vi "Get SMO HELP.vi"(8 "error in (no error)":errorcluster, 10 "Command":string, 11 "Inst.FP in":refnum<class "Inst.FP.lvclass">) -> (0 "error out":errorcluster, 2 "help cluster":T1, 3 "Inst.FP out":refnum<class "Inst.FP.lvclass">)   [LabVIEW 2019, in "Inst.FP.lvclass"]
uses:
  Inst.FP.lvclass
  <userlib>/LevyLab/Instrument Framework/subsystems/Help/typedefs/Help--cluster.ctl
  Typedefs/Inst.FP.Commands--Enum.ctl
  Typedefs/Inst.FP.pushButton--Cluster.ctl
  Typedefs/Inst.FP.Buttons--Enum.ctl
  Typedefs/Inst.FP.setMode--Cluster.ctl
  Typedefs/Inst.FP.Modes--Enum.ctl
  Typedefs/Inst.FP.getMode--Cluster.ctl
  <userlib>/LevyLab/Instrument Framework/Instrument Types/Cryostat/Instrument.Cryostat.lvclass
  <userlib>/LevyLab/Instrument Framework/subsystems/Help/Help.lvclass
  <userlib>/LevyLab/Instrument Framework/Instrument/Typedefs/Instrument.Commands--Enum.ctl
  <userlib>/LevyLab/Instrument Framework/Instrument/Instrument.lvclass
  <userlib>/LevyLab/Instrument Framework/Instrument/Typedefs/Instrument.IDN--cluster.ctl
  <vilib>/PRIrvin/JSON-Schema/JSON-Schema.lvlib
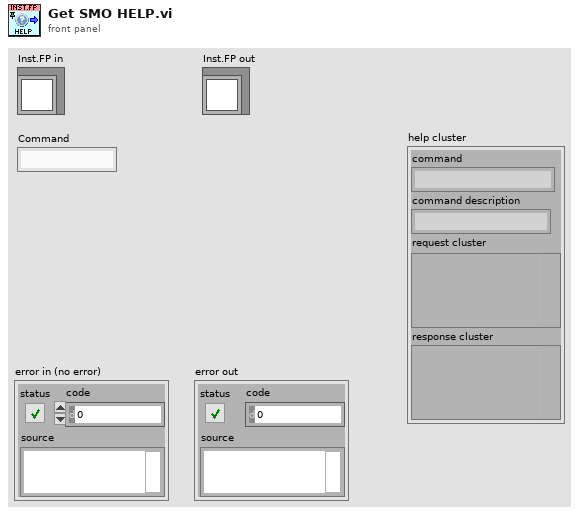
[diagram p1: front panel]
types:
  T1 = typedef "Instrument.lvlib/Help.lvclass/Help--cluster.ctl" = cluster{"command":string, "command description":string, "request cluster":variant, "response cluster":variant}
  T2 = typedef "Inst.FP.lvclass/Inst.FP.pushButton--Cluster.ctl" = cluster{"Button":T3}
  T3 = typedef "Inst.FP.lvclass/Inst.FP.Buttons--Enum.ctl" = enum16{"Start", "3He", "4He", "Normal", "Recovery", "Auto", "LED Test", "Reset"}
  T4 = typedef "Inst.FP.lvclass/Inst.FP.setMode--Cluster.ctl" = cluster{"Mode":T5}
  T5 = typedef "Inst.FP.lvclass/Inst.FP.Modes--Enum.ctl" = enum16{"AUTO MODE OFF", "START", "CONDENSING 3He", "CONDENSING 4He", "NORMAL CIRCULATION", "RECOVERY OF THE MIXTURE", "RECOVERY: BLOCKAGE or OVERPRESSURE"}
  T6 = typedef "Inst.FP.lvclass/Inst.FP.getMode--Cluster.ctl" = cluster{"Mode":T5}
  T7 = typedef "Instrument.lvlib/Instrument.lvclass/Instrument.Commands--Enum.ctl" = enum16{"ACK", "HELP", "IDN", "getAll", "getAllData"}
  T8 = typedef "Instrument.lvlib/Instrument.lvclass/Instrument.IDN--cluster.ctl" = cluster{"vendor":string, "model":string, "serial":string, "firmware":string}
  T9 = typedef "Inst.FP.lvclass/Inst.FP.Commands--Enum.ctl" = enum16{"getMode", "setMode", "pushButton"}
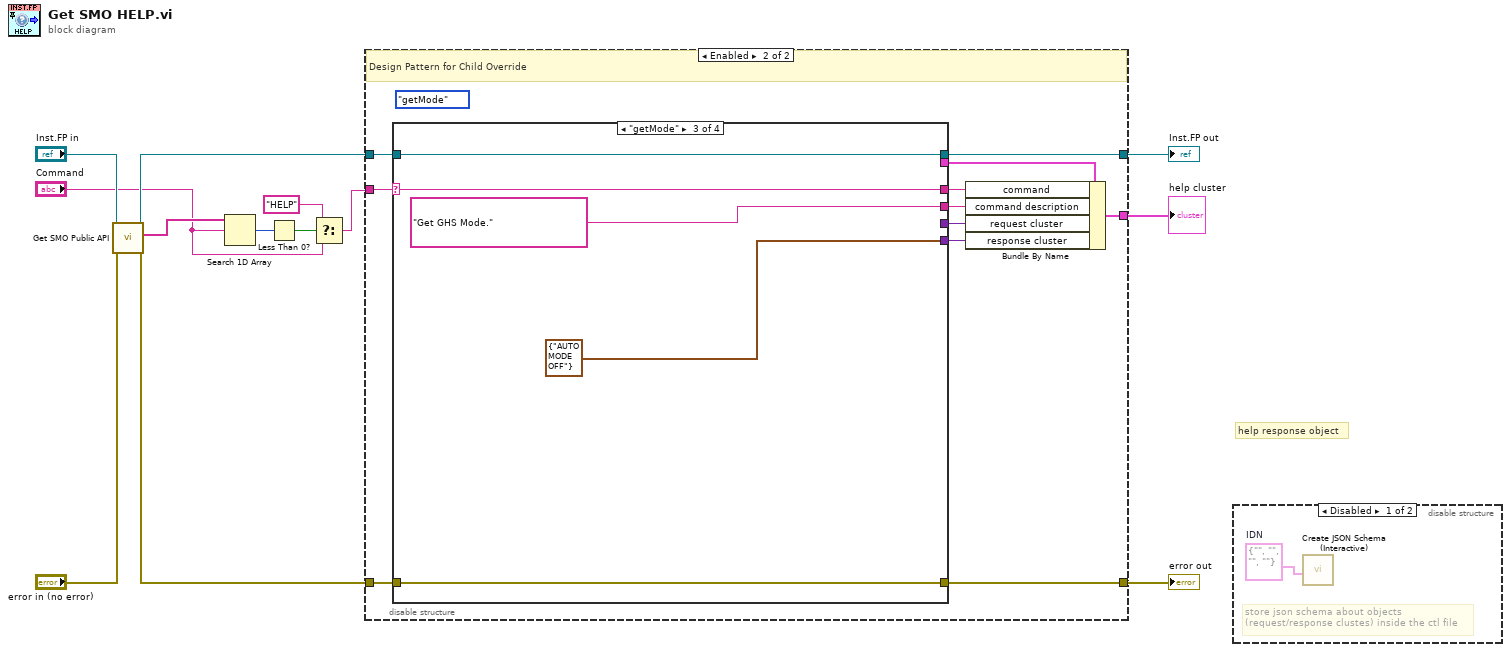
[diagram p0: block diagram]
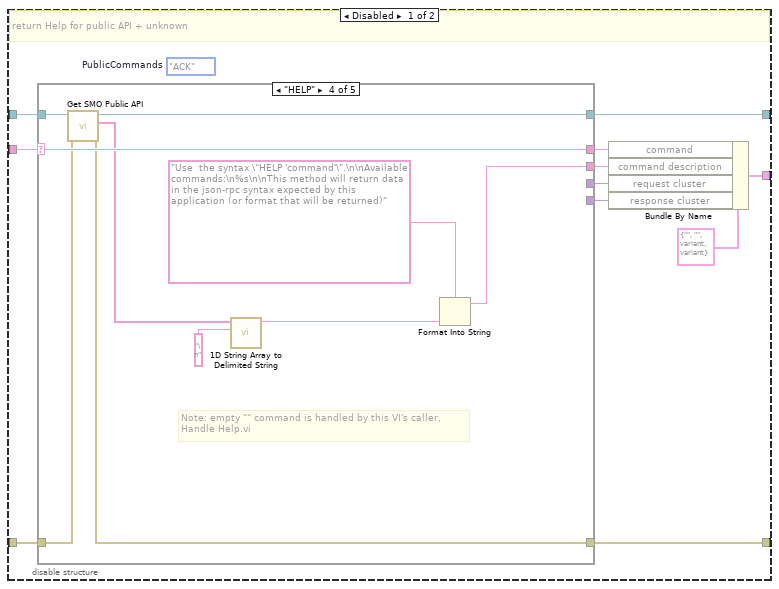
[diagram p2: hidden frame]
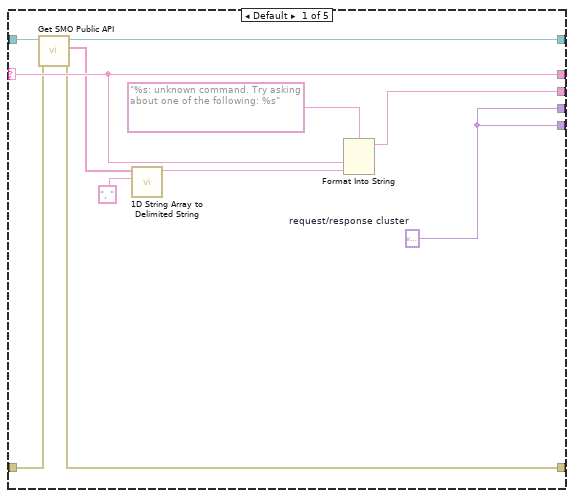
[diagram p3: hidden frame]
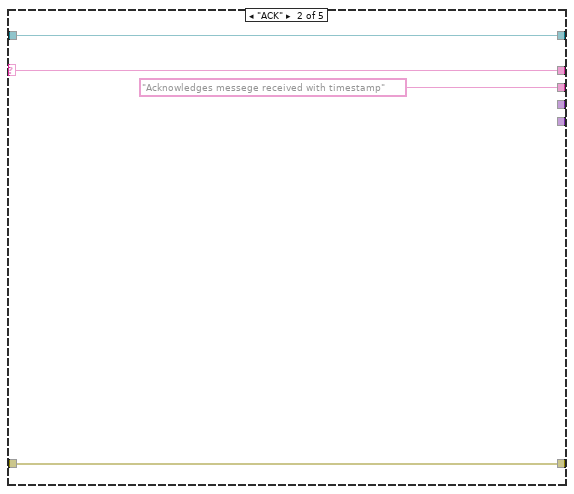
[diagram p4: hidden frame]
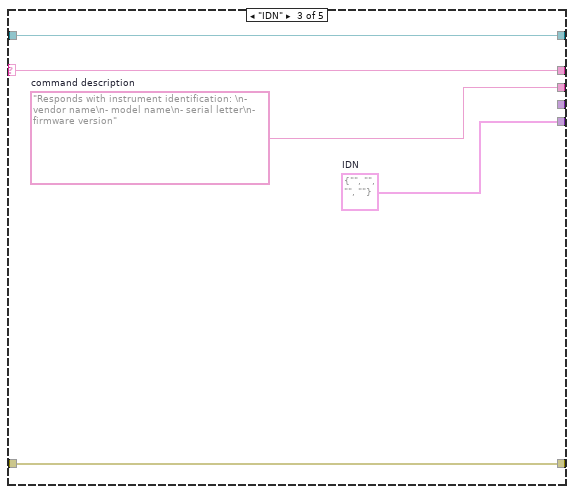
[diagram p5: hidden frame]
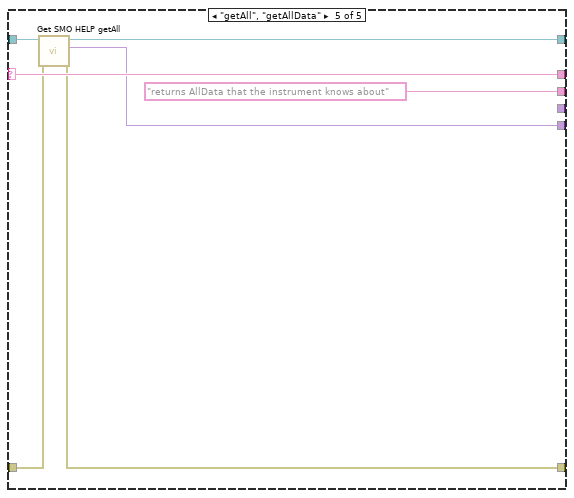
[diagram p6: hidden frame]
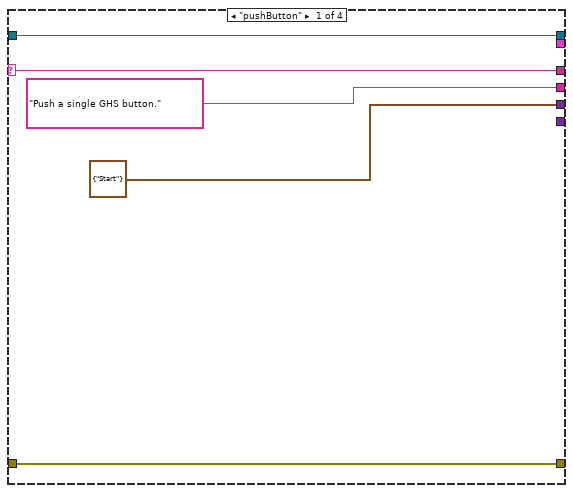
[diagram p7: hidden frame]
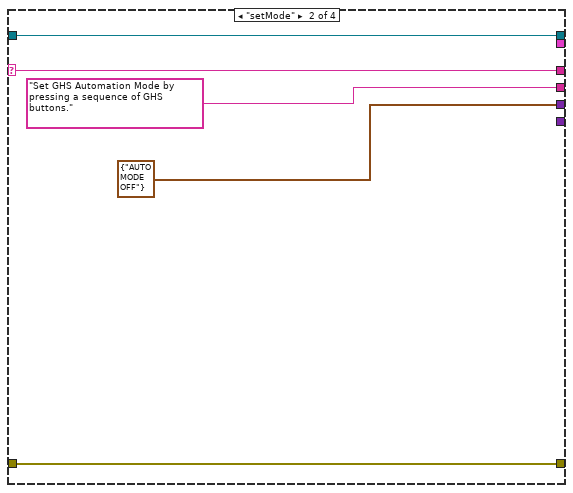
[diagram p8: hidden frame]
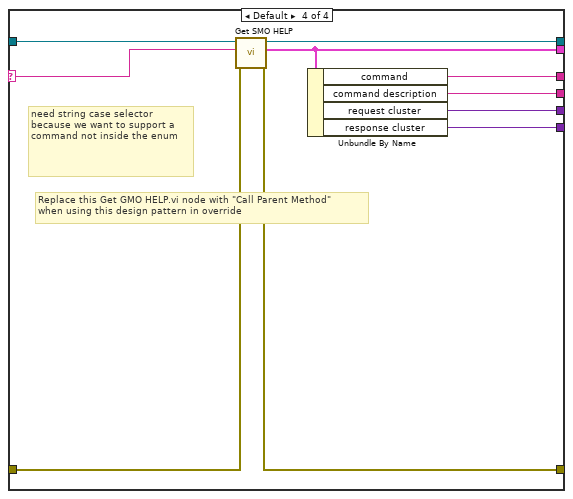
[diagram p9: hidden frame]
diagram:
  # "help response object"
  n1 = call-dynamic "Get SMO Public API.vi"("error in (no error)"="error in (no error)", "Inst.FP in"="Inst.FP in") -> ("error out"=w7:errorcluster, "Commands"=w3:string[], "Inst.FP out"=w9:refnum<class "Inst.FP.lvclass">)  [unwired: 7 in]
  n2 = Search 1D Array(1D array=w3, element="Command") -> (index of element=w6:i32)  [unwired: 1 in]
  n3 = Less Than 0?(x=w6) -> (x < 0?=w5:bool)
  n4 = Select(t="HELP", s=w5, f="Command") -> (s? t:f=w1:string)
  n5 = disable-structure shown="Enabled" {
    disable-tunnel: [w24 w64] -> w13
    disable-tunnel: w9 -> [w23 w65]
    disable-tunnel: w7 -> [w22 w70]
    disable-tunnel: [w18 w72] -> w11
    disable-tunnel: [w15 w71] -> w12
    disable-tunnel: w1 -> [w14 w62]
    frame Disabled {
      (unwired) Instrument.Commands--Enum."ACK"  # PublicCommands
      # "return Help for public API + unknown"
      n6 = case shown="\"HELP\"" w14 {
        selector: w14 -> [w31 w37 w43 w51 w60]
        tunnel: w22 -> [w28 w39 w41 w48 w59]
        tunnel: [w29 w39 w41 w49 w58] -> w18
        tunnel: [w33 "Acknowledges messege received with timestamp" w44 w45 "returns AllData that the instrument knows about"] -> w20
        tunnel: [w26 _ _ _ _] -> w19
        tunnel: [w26 _ w40 _ w55] -> w17
        tunnel: [w31 w37 w43 w51 w60] -> w21
        tunnel: w23 -> [w30 w36 w42 w50 w56]
        tunnel: [w27 w36 w42 w47 w57] -> w24
        frame Default {
          w26 = variant  # request/response cluster
          n7 = call-dynamic "Get SMO Public API.vi"("error in (no error)"=w28, "Inst.FP in"=w30) -> ("error out"=w29:errorcluster, "Commands"=w25:string[], "Inst.FP out"=w27:refnum<class "Inst.FP.lvclass">)  [unwired: 7 in]
          n8 = call <vilib>:"1D String Array to Delimited String.vi"("delimiter"=", ", "string array"=w25) -> ("delimited string"=w34:string)  [unwired: 9 in]
          n9 = Format Into String(format string="%s: unknown command. Try asking about one of the following: %s", w31, w34) -> (resulting string=w33:string)  [unwired: 2 in, 1 out]
        }
        frame "ACK" {
        }
        frame "IDN" {
          w40 = T8 {"vendor"="", "model"="", "serial"="", "firmware"=""}  # IDN
          w44 = "Responds with instrument identification: \n- vendor name\n- model name\n- serial letter\n- firmware version"  # command description
        }
        frame "HELP" {
          # "Note: empty \"\" command is handled by this VI's caller,\nHandle Help.vi"
          n10 = call-dynamic "Get SMO Public API.vi"("error in (no error)"=w48, "Inst.FP in"=w50) -> ("error out"=w49:errorcluster, "Commands"=w46:string[], "Inst.FP out"=w47:refnum<class "Inst.FP.lvclass">)  [unwired: 7 in]
          n11 = call <vilib>:"1D String Array to Delimited String.vi"("delimiter"="\n", "string array"=w46) -> ("delimited string"=w54:string)  [unwired: 9 in]
          n12 = Format Into String(format string="Use  the syntax \"HELP 'command'\".\n\nAvailable commands:\n%s\n\nThis method will return data in the json-rpc syntax expected by this application (or format that will be returned)", w54) -> (resulting string=w45:string)  [unwired: 2 in, 1 out]
        }
        frame "getAll", "getAllData" {
          n13 = call-dynamic "Get SMO HELP getAll.vi"("error in (no error)"=w59, "Inst.FP in"=w56) -> ("error out"=w58:errorcluster, "response cluster"=w55:variant, "Inst.FP out"=w57:refnum<class "Inst.FP.lvclass">)  [unwired: 7 in]
        }
      }
      n14 = Bundle By Name(cluster=T1 {"command"="", "command description"="", "request cluster"=variant, "response cluster"=variant} ("Help"), "command"=w21, "command description"=w20, "request cluster"=w19, "response cluster"=w17) -> (w15:T1)
    }
    frame Enabled {
      (unwired) Inst.FP.Commands--Enum."getMode" ("Commands")
      # "Design Pattern for Child Override"
      n15 = case shown="\"getMode\"" w62 {
        selector: w62 -> [w77 w82 w87 w96]
        tunnel: [w77 w82 w87 w91] -> w69
        tunnel: w70 -> [w76 w81 w86 w89]
        tunnel: [w76 w81 w86 w88] -> w72
        tunnel: ["Push a single GHS button." "Set GHS Automation Mode by pressing a sequence of GHS buttons." "Get GHS Mode." w92] -> w68
        tunnel: [T2 {"Button"=enum."Start"} ("pushButton") T4 {"Mode"=enum."AUTO MODE OFF"} ("setMode") _ w93] -> w67
        tunnel: [_ _ T6 {"Mode"=enum."AUTO MODE OFF"} ("getMode") w94] -> w66
        tunnel: w65 -> [w74 w79 w84 w97]
        tunnel: [w74 w79 w84 w95] -> w64
        tunnel: [_ _ _ w90] -> w63
        frame "pushButton" {
        }
        frame "setMode" {
        }
        frame "getMode" {
        }
        frame Default {
          # "need string case selector because we want to support a command not inside the enum"
          # "Replace this Get GMO HELP.vi node with \"Call Parent Method\"\nwhen using this design pattern in override"
          n16 = call-parent "Get SMO HELP.vi"("error in (no error)"=w89, "Command"=w96, "Instrument.Cryostat in"=w97) -> ("error out"=w88:errorcluster, "help cluster"=w90:T1, "Instrument.Cryostat out"=w95:refnum<class "Inst.FP.lvclass">)  [unwired: 6 in]
          n17 = Unbundle By Name(w90) -> ("command"=w91:string, "command description"=w92:string, "request cluster"=w93:variant, "response cluster"=w94:variant)
        }
      }
      n18 = Bundle By Name(cluster=w63, "command"=w69, "command description"=w68, "request cluster"=w67, "response cluster"=w66) -> (w71:T1)
    }
  }
  "Inst.FP out" <- w13
  "help cluster" <- w12
  "error out" <- w11
  n19 = disable-structure shown="Disabled" {
    frame Disabled {
      w98 = T8 {"vendor"="", "model"="", "serial"="", "firmware"=""}  # IDN
      # "store json schema about objects\n(request/response clustes) inside the ctl file"
      n20 = call <vilib>:"Create JSON Schema (Interactive).vi"("LV Object"=w98) -> ()  [unwired: 9 in, 2 out]
    }
    frame Enabled {
    }
  }
